vi "nominal channel set metadata.vi"(0 "client":i32, 1 "description":string, 2 "clear_unit":bool, 5 "data_source_rid":string, 7 "name":string, 9 "data_type":i32, 11 "error in (no error)":errorcluster, 12 "unit":string, 13 "out_channel":i32) -> (4 "out_channel out":i32, 6 "function return":i32, 15 "error out":errorcluster)   [LabVIEW 2020, in "client.lvlib"]
doc: "int32_t nominal_channel_set_metadata(int32_t client,\n const char *data_source_rid,\n const char *name,\n int32_t data_type,\n const char *description,\n const char *unit,\n bool clear_unit,\n int32_t *out_channel);"
uses:
  client.lvlib
  bin/nominalClient_64.dll
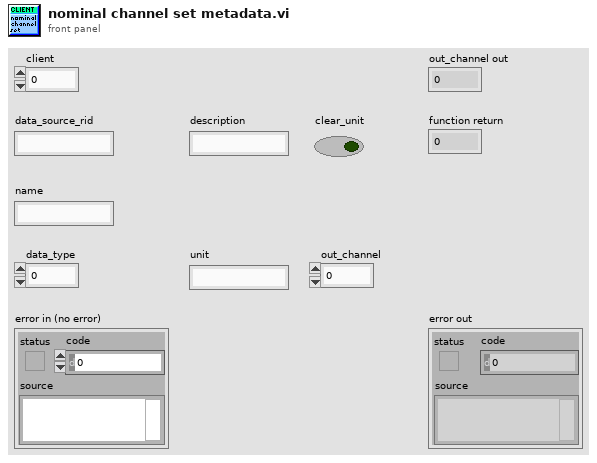
[diagram p1: front panel]
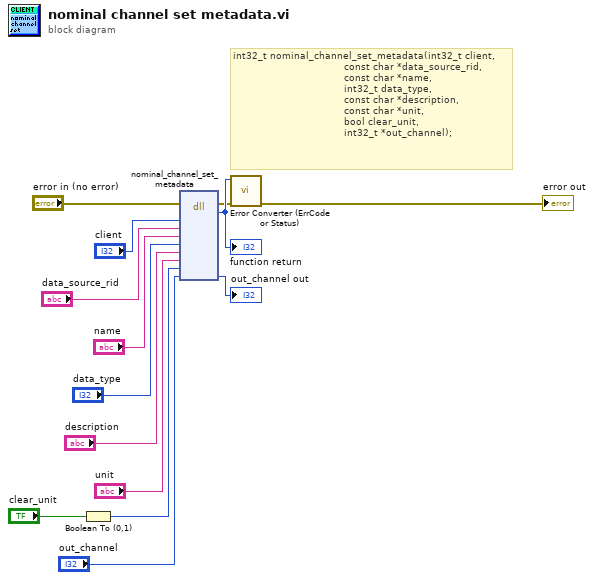
[diagram p0: block diagram]
diagram:
  # "int32_t nominal_channel_set_metadata(int32_t client,\n                                     const char *data_source_rid,\n                                     const char *name,\n                                     int32_t data_type,\n                                     const char *description,\n                                     const char *unit,\n                                     bool clear_unit,\n                                     int32_t *out_channel);"
  n1 = Boolean To (0,1)(Boolean="clear_unit") -> (0, 1=w6:i16)
  n2 = dll-call lib="C:/code/labview-client-rs/lv_src/bin/nominalClient_*.*" fn="nominal_channel_set_metadata"(error in="error in (no error)", "client"="client", "data_source_rid"="data_source_rid", "name"="name", "data_type"="data_type", "description"="description", "unit"="unit", "clear_unit"=w6, "out_channel"="out_channel") -> (error out=w2:errorcluster, w14:i32, "out_channel"=→"out_channel out":i32)  [unwired: 9 in, 1 out]
  "function return" <- w14
  n3 = call "Error Converter (ErrCode or Status).vi"("error in (no error)"=w2, "error code"=w14) -> ("error out"=→"error out":errorcluster)  [unwired: 9 in]
